vi "Project explorer Navigation.vi"(11 "Data Cluster":T1) -> (0 "error out":errorcluster)   [LabVIEW 2019, in "Panther Dashboard.lvlib"]
uses:
  Panther Dashboard.lvlib
  <vilib>/National Instruments/Tree Map/Tree Map Data.ctl
  <vilib>/National Instruments/Tree Map/Tree Map.lvlib
  Maps List and refs--cluster.ctl
  Module type--enum.ctl
  Project References--cluster.ctl
  DQMH Modules Info--cluster.ctl
  Module Data--cluster.ctl
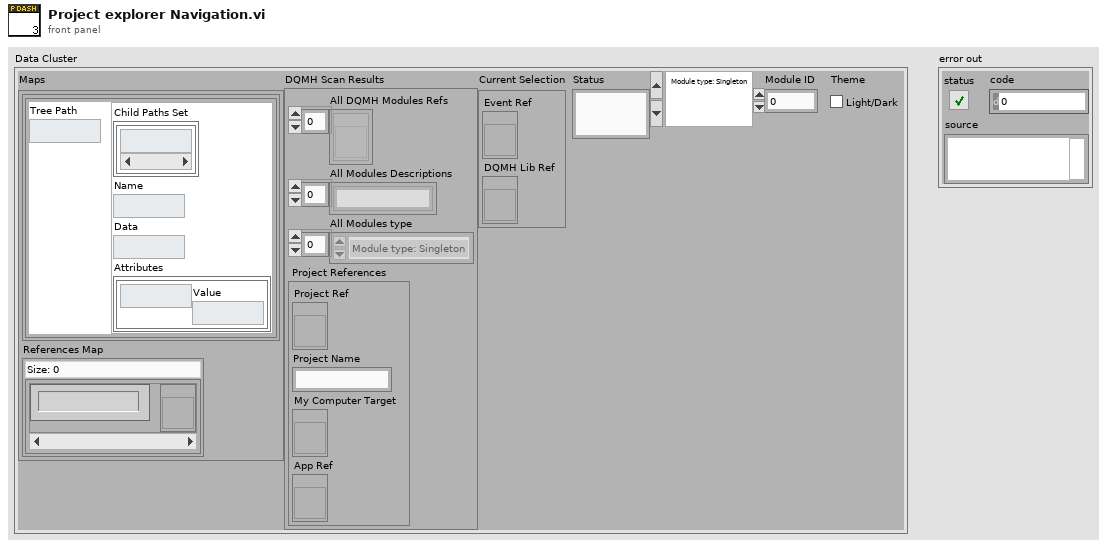
[diagram p1: front panel]
types:
  T1 = typedef "Panther Dashboard.lvlib/Module Data--cluster.ctl" = cluster{"Maps":T2, "DQMH Scan Results":T4, "Current Selection":cluster{"Event Ref":refnum<vi>, "DQMH Lib Ref":refnum<vi>}, "Status":string, "Module type":T5, "Module ID":i32, "Theme":bool}
  T2 = typedef "Panther Dashboard.lvlib/Maps List and refs--cluster.ctl" = cluster{"Tree Map":T3, "References Map":map{string, refnum<vi>}}
  T3 = typedef "Tree Map.lvlib/Tree Map Data.ctl" = map{string, cluster{"Child Paths Set":set{string}, "Name":string, "Data":string, "Attributes":map{string, string}}}
  T4 = typedef "Panther Dashboard.lvlib/DQMH Modules Info--cluster.ctl" = cluster{"All DQMH Modules Refs":refnum<vi>[], "All Modules Descriptions":string[], "All Modules type":T5[], "Project References":T6}
  T5 = typedef "Panther Dashboard.lvlib/Module type--enum.ctl" = enum16{"Module type: Singleton", "Module type: Cloneable"}
  T6 = typedef "Panther Dashboard.lvlib/Project References--cluster.ctl" = cluster{"Project Ref":refnum<vi>, "Project Name":string, "My Computer Target":refnum<vi>, "App Ref":refnum<vi>}
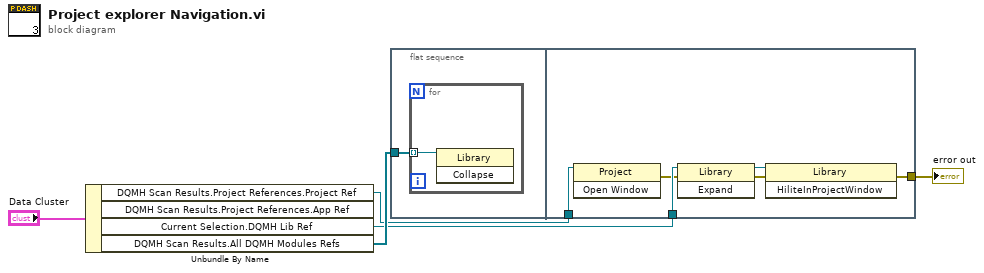
[diagram p0: block diagram]
diagram:
  n1 = Unbundle By Name("Data Cluster") -> ("DQMH Scan Results.Project References.Project Ref"=w2:refnum<vi>, "Current Selection.DQMH Lib Ref"=w3:refnum<vi>, "DQMH Scan Results.All DQMH Modules Refs"=w5:refnum<vi>[])  [unwired: 1 out]
  n2 = flat-sequence {
    tunnel: w5 -> [w6]
    tunnel: w3 -> [w13]
    tunnel: w2 -> [w12]
    tunnel: [w11] -> w1
    frame #0 {
      n3 = for {
        tunnel: w6 -> [w7] mode=indexing
        n4 = invoke class="Library" method="Collapse"(reference=w7) -> ()  [unwired: 2 in, 3 out]
      }
    }
    frame #1 {
      n5 = invoke class="Project" method="Open Window"(reference=w12) -> (error out=w10:errorcluster)  [unwired: 2 in, 2 out]
      n6 = invoke class="Library" method="Expand"(reference=w13, error in=w10) -> (reference out=w8:refnum<vi>, error out=w9:errorcluster)  [unwired: 1 in, 1 out]
      n7 = invoke class="Library" method="HiliteInProjectWindow"(reference=w8, error in=w9) -> (error out=w11:errorcluster)  [unwired: 1 in, 2 out]
    }
  }
  "error out" <- w1
